vi "INIT Load Database.vi"(8 "error in (no error)":errorcluster) -> (0 "error out":errorcluster, 2 "cancelled":bool, 3 "DB Alias data":T1)   [LabVIEW 2018, in "CAN Gateway System Explorer.lvlib"]
uses:
  CAN Gateway System Explorer.lvlib
  Types/Alias DB data.ctl
panel:
  in  "Open Button":bool
  in  "Cancel Button":bool
  in  "OK Button":bool
  in  "Existing Aliases":string(combo)
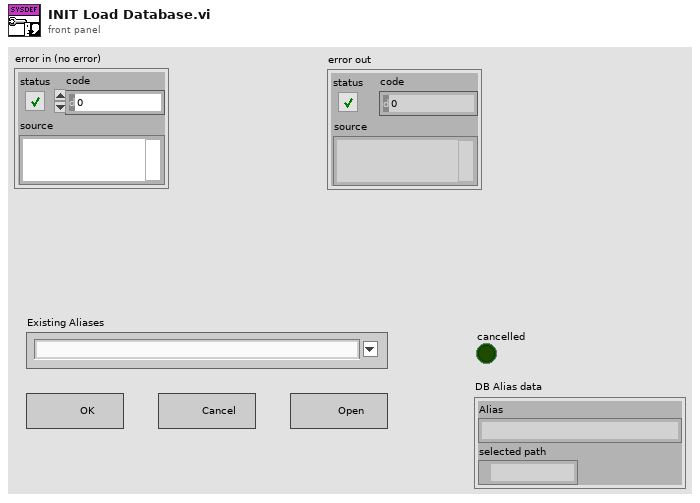
[diagram p1: front panel]
types:
  T1 = typedef "CAN Gateway System Explorer.lvlib/Alias DB data.ctl" = cluster{"Alias":string, "selected path":path}
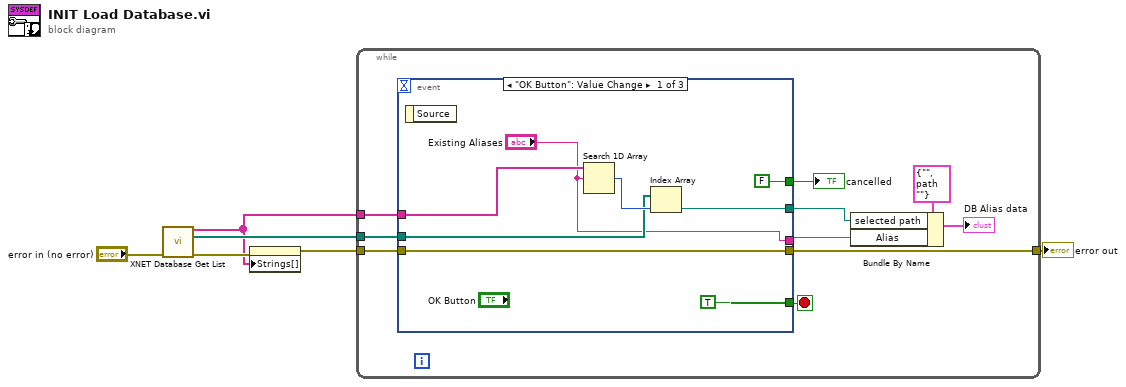
[diagram p0: block diagram]
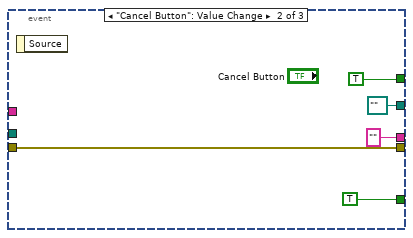
[diagram p2: hidden frame]
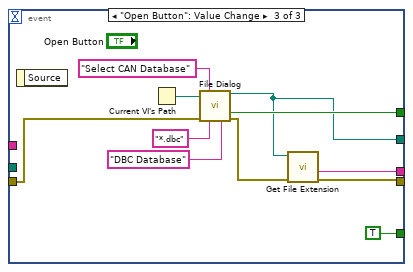
[diagram p3: hidden frame]
diagram:
  n1 = call <vilib>:"XNET Database Get List.vi"("error in (no error)"="error in (no error)") -> ("array of alias"=w1:string[], "array of filepath"=w2:path[], "error out"=w6:errorcluster)  [unwired: 12 in]
  n2 = property on="Existing Aliases" class="CmbBox"(error in=w6, "Strings[]"=w1) -> (error out=w3:errorcluster)  [unwired: 1 in, 1 out]
  n3 = while {
    tunnel: [w16] -> w5
    tunnel: w3 -> [w14]
    tunnel: w2 -> [w12]
    tunnel: w1 -> [w11]
    stop <- w15 stop-if-true
    n4 = event shown="[0] \"OK Button\": Value Change" {
      selector: _ -> [_ _ _]
      dyn-events: _ -> [_ _ _]
      timeout: _ -> [_ _ _]
      tunnel: [w19 w28 w34] -> w16
      tunnel: [TRUE TRUE TRUE] -> w15
      tunnel: w14 -> [w19 w28 w36]
      tunnel: [FALSE ("cancelled") TRUE w37] -> w13
      tunnel: ["Existing Aliases" "" ("filename without extension") w33] -> w7
      tunnel: [w18 path "" ("selected path") w30] -> w8
      tunnel: w12 -> [w20 _ _]
      tunnel: w11 -> [w22 _ _]
      event "OK Button": Value Change {
        n5 = event-data() -> ()  [unwired: 1 in, 1 out]
        n6 = Search 1D Array(1D array=w22, element="Existing Aliases") -> (index of element=w21:i32)  [unwired: 1 in]
        n7 = Index Array(array=w20, index=w21) -> (element=w18:path)
      }
      event "Cancel Button": Value Change {
        n8 = event-data() -> ()  [unwired: 1 in, 1 out]
      }
      event "Open Button": Value Change {
        n9 = event-data() -> ()  [unwired: 1 in, 1 out]
        n10 = Current VI's Path() -> (path=w31:path)
        n11 = call "File Dialog"("start path"=w31, "prompt"="Select CAN Database", "error in"=w36, "pattern (all files)"="*.dbc", "pattern label"="DBC Database") -> ("selected path"=w30:path, "cancelled"=w37:bool, "error out"=w35:errorcluster)  [unwired: 7 in, 1 out]
        n12 = call <vilib>:"Get File Extension.vi"("error in (no error)"=w35, "file"=w30) -> ("error out"=w34:errorcluster, "filename without extension"=w33:string)  [unwired: 5 in, 3 out]
      }
    }
    "cancelled" <- w13
    n13 = Bundle By Name(cluster=T1 {"Alias"="", "selected path"=path ""} ("DB Alias data"), "selected path"=w8, "Alias"=w7) -> (→"DB Alias data":T1)
  }
  "error out" <- w5
